vi "Capture_Tab.vi"(9 "vi path":path=path "D:/Falcon_char/Labview Files/Falcon_ADC_INL_DNL_SNR_GUI.vi", 10 "Select Tab":i32, 11 "path to JPEG file":path) -> (3 "Tab Name":string)   [LabVIEW 2016]
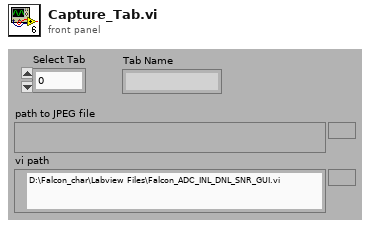
[diagram p1: front panel]
types:
  T1 = typedef "imagedata.ctl" = cluster{"image type":i32, "image depth":i32, "image":u8[], "mask":u8[], "colors":u32[], "Rectangle":cluster{"left":i16, "top":i16, "right":i16, "bottom":i16}}
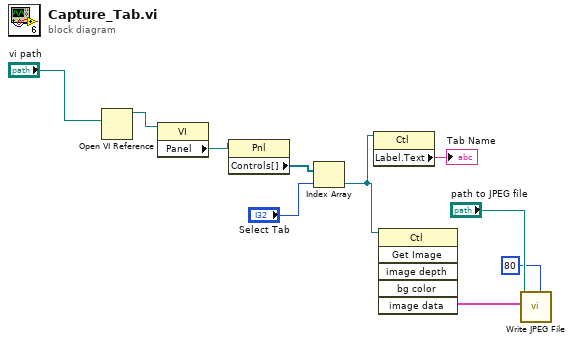
[diagram p0: block diagram]
diagram:
  n1 = Open VI Reference(vi path="vi path") -> (vi reference=w9:refnum<vi>)  [unwired: 5 in, 1 out]
  n2 = property class="VI"(reference=w9) -> ("Panel"=w8:refnum<vi>)  [unwired: 1 in, 2 out]
  n3 = property class="Pnl"(reference=w8) -> ("Controls[]"=w7:refnum<vi>[])  [unwired: 1 in, 2 out]
  n4 = Index Array(array=w7, index="Select Tab") -> (element=w5:refnum<vi>)
  n5 = property class="Ctl"(reference=w5) -> ("Label.Text"=→"Tab Name":string)  [unwired: 1 in, 2 out]
  n6 = invoke class="Ctl" method="Get Image"(reference=w5) -> ("image data"=w3:T1)  [unwired: 5 in, 5 out]
  n7 = call <vilib>:"Write JPEG File.vi"("quality (80)"=80, "image data"=w3, "path to JPEG file"="path to JPEG file") -> ()  [unwired: 7 in, 2 out]
